vi "tag bus to parameters.vi"(9 "indices":T1, 11 "tag bus in":T3) -> (2 "data cluster":T2, 3 "tag bus out":T3)   [LabVIEW 2013, in "Temperature Controller Logic runtime.lvclass"]
uses:
  Temperature Controller Logic runtime.lvclass
  <vilib>/NI/Tag Bus/table/data table.ctl
  parameter user data.ctl
  configuration/parameter data indices.ctl
  <vilib>/NI/Tag Bus/table/data polymorphs/read one/read Boolean.vi
  <vilib>/NI/Tag Bus/table/data polymorphs/read one/read Double.vi
  <vilib>/NI/Tag Bus/table/data table.lvlib
  configuration/Temperature Controller Logic configuration.lvclass
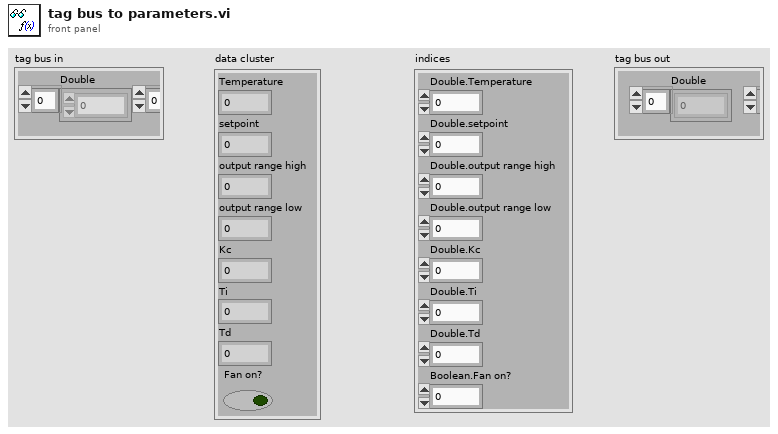
[diagram p1: front panel]
types:
  T1 = typedef "Temperature Controller Logic configuration.lvclass/parameter data indices.ctl" = cluster{"Double.Temperature":i32, "Double.setpoint":i32, "Double.output range high":i32, "Double.output range low":i32, "Double.Kc":i32, "Double.Ti":i32, "Double.Td":i32, "Boolean.Fan on?":i32}
  T2 = typedef "Temperature Controller Logic runtime.lvclass/parameter user data.ctl" = cluster{"Temperature":dbl, "setpoint":dbl, "output range high":dbl, "output range low":dbl, "Kc":dbl, "Ti":dbl, "Td":dbl, "Fan on?":bool}
  T3 = typedef "tag bus.lvlib/data table.lvlib/data table.ctl" = cluster{"Double":dbl[], "Single":sgl[], "I64":i64[], "I32":i32[], "I16":i16[], "I8":i8[], "U64":u64[], "U32":u32[], "U16":u16[], "U8":u8[], "Boolean":bool[], "String":string[], "Array of Double":cluster{"DBL Array":dbl[]}[], "Array of Single":cluster{"SGL Array":sgl[]}[], "Array of I64":cluster{"I64 Array":i64[]}[], "Array of I32":cluster{"I32 Array":i32[]}[], "Array of I16":cluster{"I16 Array":i16[]}[], "Array of I8":cluster{"I8 Array":i8[]}[], "Array of U64":cluster{"U64 Array":u64[]}[], "Array of U32":cluster{"U32 Array":u32[]}[], "Array of U16":cluster{"U16 Array":u16[]}[], "Array of U8":cluster{"U8 Array":u8[]}[], "Array of Boolean":cluster{"Boolean Array":bool[]}[], "Array of String":cluster{"String Array":string[]}[]}
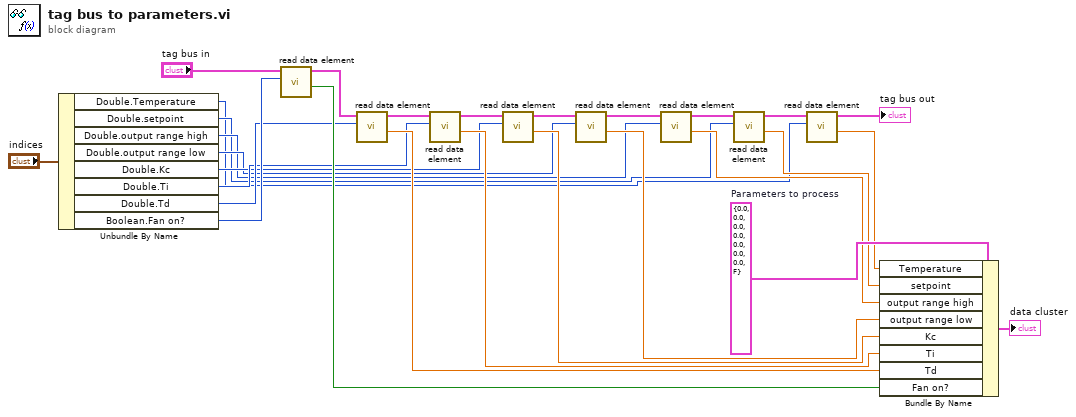
[diagram p0: block diagram]
diagram:
  w27 = T2 {"Temperature"=0.0, "setpoint"=0.0, "output range high"=0.0, "output range low"=0.0, "Kc"=0.0, "Ti"=0.0, "Td"=0.0, "Fan on?"=FALSE}  # Parameters to process
  n1 = Unbundle By Name("indices") -> ("Double.Temperature"=w2:i32, "Double.setpoint"=w5:i32, "Double.output range high"=w8:i32, "Double.output range low"=w11:i32, "Double.Kc"=w14:i32, "Double.Ti"=w17:i32, "Double.Td"=w20:i32, "Boolean.Fan on?"=w23:i32)
  n2 = call-poly <vilib>:"read data element.vi"("index"=w23, "data table in"="tag bus in") -> ("value"=w24:bool, "data table out"=w22:T3)  [unwired: 8 in]
  n3 = call-poly <vilib>:"read data element.vi"("index"=w20, "data table in"=w22) -> ("value"=w21:dbl, "data table out"=w19:T3)  [unwired: 8 in]
  n4 = call-poly <vilib>:"read data element.vi"("index"=w17, "data table in"=w19) -> ("value"=w18:dbl, "data table out"=w16:T3)  [unwired: 8 in]
  n5 = call-poly <vilib>:"read data element.vi"("index"=w14, "data table in"=w16) -> ("value"=w15:dbl, "data table out"=w13:T3)  [unwired: 8 in]
  n6 = call-poly <vilib>:"read data element.vi"("index"=w11, "data table in"=w13) -> ("value"=w12:dbl, "data table out"=w10:T3)  [unwired: 8 in]
  n7 = call-poly <vilib>:"read data element.vi"("index"=w8, "data table in"=w10) -> ("value"=w9:dbl, "data table out"=w7:T3)  [unwired: 8 in]
  n8 = call-poly <vilib>:"read data element.vi"("index"=w5, "data table in"=w7) -> ("value"=w6:dbl, "data table out"=w4:T3)  [unwired: 8 in]
  n9 = call-poly <vilib>:"read data element.vi"("index"=w2, "data table in"=w4) -> ("value"=w3:dbl, "data table out"=→"tag bus out":T3)  [unwired: 8 in]
  n10 = Bundle By Name(cluster=w27, "Temperature"=w3, "setpoint"=w6, "output range high"=w9, "output range low"=w12, "Kc"=w15, "Ti"=w18, "Td"=w21, "Fan on?"=w24) -> (→"data cluster":T2)
